vi "Variant to Type ID.vi"(11 "Variant":variant) -> (3 "Type ID":string, 5 "Skip?":bool)   [LabVIEW 2020, in "Better Search.lvlib"]
uses:
  Better Search.lvlib
  <vilib>/Utility/Data Type/Type Definitions/Data Type.ctl
  <vilib>/Utility/Data Type/NI_Data Type.lvlib
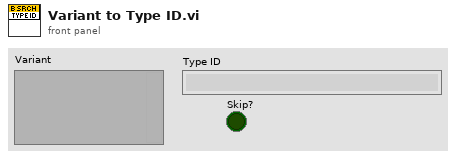
[diagram p1: front panel]
types:
  T1 = typedef "NI_Data Type.lvlib/Data Type.ctl" = enum8{"Invalid Type", "Void", "I8", "I16", "I32", "I64", "U8", "U16", "U32", "U64", "Single Float", "Double Float", "Extended Float", "Single Complex", "Double Complex", "Extended Complex", "Enum U8", "Enum U16", "Enum U32", "Enum U64", "Single Float With Unit", "Double Float With Unit", "Extended Float With Unit", "Single Complex with Unit", "Double Complex with Unit", "Extended Complex with Unit", "Boolean", "String", "Path", "Picture", "Tag", "Array", "Cluster", "Variant", "LV Variant", "Waveform", "Timestamp", "Digital Waveform", "Digital Data", "ExpressData", "Refnum", "External Data", "VI", "Poly VI", "LabVIEW Class Instance", "Fixed Point", "Set Collection", "Map Collection"}
  T2 = typedef "NI_Data Type.lvlib/Type Definition Info.ctl" = cluster{"Name":string, "Timestamp":u32}
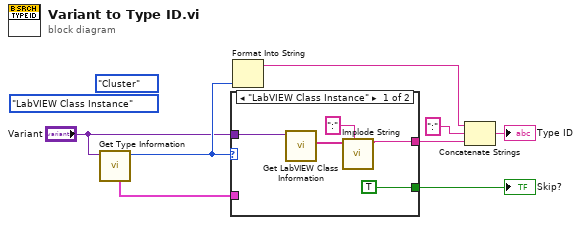
[diagram p0: block diagram]
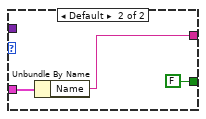
[diagram p2: hidden frame]
diagram:
  (unwired) Data_Type."LabVIEW Class Instance" ("type")
  (unwired) Data_Type."Cluster" ("type")
  n1 = call <vilib>:"Get Type Information.vi"("variant"="Variant") -> ("type"=w8:T1, "type definition info"=w4:T2)  [unwired: 6 in, 3 out]
  n2 = case shown="\"LabVIEW Class Instance\"" w8 {
    tunnel: "Variant" -> [w13 _]
    tunnel: [w9 w15] -> w7
    tunnel: w4 -> [_ w16]
    tunnel: [TRUE FALSE] -> w1
    frame "LabVIEW Class Instance" {
      n3 = call <vilib>:"Get LabVIEW Class Information.vi"("variant"=w13) -> ("qualified LabVIEW class name"=w11:string[])  [unwired: 8 in, 2 out]
      n4 = call "Implode String.vi"("Delimiter (Comma)"=":" ("delimiter"), "String Array"=w11) -> ("Delimited String"=w9:string)  [unwired: 9 in]
    }
    frame Default {
      n5 = Unbundle By Name(w16) -> ("Name"=w15:string)
    }
  }
  "Skip?" <- w1
  n6 = Format Into String(w8) -> (resulting string=w5:string)  [unwired: 3 in, 1 out]
  n7 = Concatenate Strings(w5, ":" ("string"), w7) -> (→"Type ID":string)
